vi "mxwScript_API_XMLTemplateNameWithOptions.vi"(8 "error in (no error)":errorcluster, 10 "wizard lock data":T1, 11 "absolutePath":string) -> (0 "error out":errorcluster, 3 "encoded absolutePath":string)   [LabVIEW 2020]
doc: "Create encoded \"absolutePath\" for adding options to the template scripting such as wizard locking."
uses:
  codeGenAPISupport.llb/cgAPI_mxwScript_WizardLockData.ctl
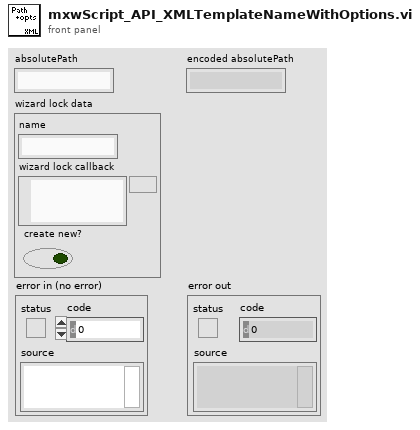
[diagram p1: front panel]
types:
  T1 = typedef "cgAPI_mxwScript_WizardLockData.ctl" = cluster{"name":string, "wizard lock callback":path, "create new?":bool}
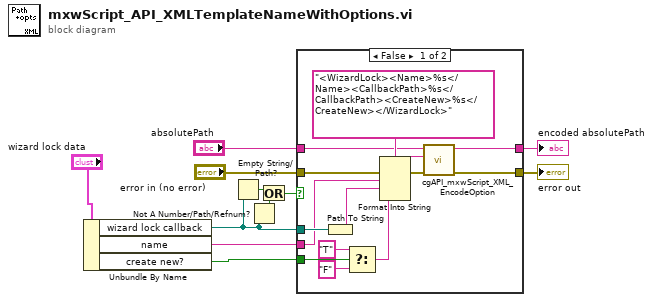
[diagram p0: block diagram]
diagram:
  n1 = Unbundle By Name("wizard lock data") -> ("wizard lock callback"=w3:path, "name"=w2:string, "create new?"=w1:bool)
  n2 = Empty String/Path?(string/path=w3) -> (empty?=w6:bool)
  n3 = Not A Number/Path/Refnum?(number/path/refnum=w3) -> (NaN/Path/Refnum?=w5:bool)
  n4 = Or(x=w6, y=w5) -> (x .or. y?=w4:bool)
  n5 = case shown="False" w4 {
    tunnel: [w25 w27] -> w11
    tunnel: [w12 w26] -> w10
    tunnel: "error in (no error)" -> [w24 w27]
    tunnel: "absolutePath" -> [w20 w26]
    tunnel: w3 -> [w19 _]
    tunnel: w2 -> [w17 _]
    tunnel: w1 -> [w16 _]
    frame False {
      n6 = Path To String(path=w19) -> (string=w18:string)
      n7 = Select(t="T", s=w16, f="F") -> (s? t:f=w13:string)
      n8 = Format Into String(format string="<WizardLock><Name>%s</Name><CallbackPath>%s</CallbackPath><CreateNew>%s</CreateNew></WizardLock>" ("control name"), error in=w24, w17, w18, w13) -> (resulting string=w21:string, error out=w23:errorcluster)  [unwired: 1 in]
      n9 = call "cgAPI_mxwScript_XML_EncodeOption.vi"("error in (no error)"=w23, "otherXML"=w21, "normalTextString"=w20) -> ("error out"=w25:errorcluster, "encodedString"=w12:string)  [unwired: 7 out]
    }
    frame True {
    }
  }
  "error out" <- w11
  "encoded absolutePath" <- w10
